vi "Compute Plot Legend Size.vi"(5 "# Plots":i32, 7 "Current Plot (Last)":i32=2147483647, 9 "Max Legend Size":i32) -> (6 "LegNumRows":u32, 8 "LegScrollVis":bool, 10 "LegScrollPos":u32)   [LabVIEW 2021, in "Graphs.lvlib"]
uses:
  Graphs.lvlib
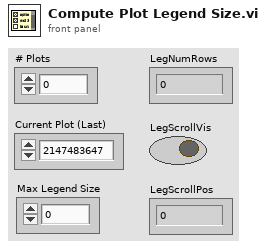
[diagram p1: front panel]
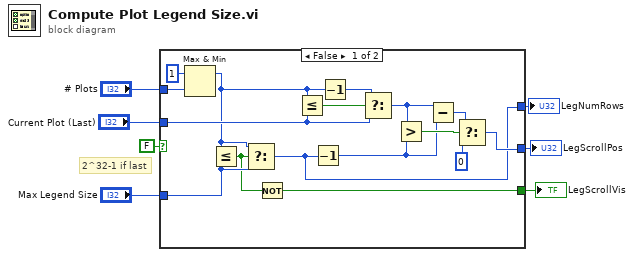
[diagram p0: block diagram]
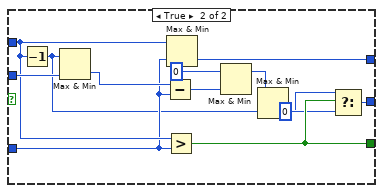
[diagram p2: hidden frame]
diagram:
  # "2^32-1 if last"
  n1 = case shown="False" FALSE {
    tunnel: [w8 w36] -> w7
    tunnel: [w9 w35] -> w6
    tunnel: [w12 w33] -> w5
    tunnel: "Current Plot (Last)" -> [w21 w32]
    tunnel: "# Plots" -> [w19 w31]
    tunnel: "Max Legend Size" -> [w16 w29]
    frame False {
      n2 = Max & Min(x=1, y=w19) -> (max(x,y)=w17:i32)  [unwired: 1 out]
      n3 = Less Or Equal?(x=w17, y=w16) -> (x <= y?=w10:bool)
      n4 = Select(t=w17, s=w10, f=w16) -> (s? t:f=w8:i32)
      n5 = Not(x=w10) -> (.not. x?=w9:bool)
      n6 = Less Or Equal?(x=w17, y=w21) -> (x <= y?=w23:bool)
      n7 = Decrement(x=w8) -> (x-1=w11:i32)
      n8 = Decrement(x=w17) -> (x-1=w22:i32)
      n9 = Select(t=w22, s=w23, f=w21) -> (s? t:f=w15:i32)
      n10 = Greater?(x=w15, y=w11) -> (0:w20:bool)
      n11 = Subtract(x=w15, y=w11) -> (x-y=w14:i32)
      n12 = Select(t=w14, s=w20, f=0) -> (s? t:f=w12:i32)
    }
    frame True {
      n13 = Decrement(x=w31) -> (x-1=w28:i32)
      n14 = Max & Min(x=w28, y=w32) -> (min(x,y)=w30:i32)  [unwired: 1 out]
      n15 = Subtract(x=w30, y=w29) -> (x-y=w24:i32)
      n16 = Greater?(x=w31, y=w29) -> (0:w35:bool)
      n17 = Max & Min(x=w31, y=w29) -> (min(x,y)=w36:i32)  [unwired: 1 out]
      n18 = Max & Min(x=0, y=w24) -> (max(x,y)=w25:i32)  [unwired: 1 out]
      n19 = Max & Min(x=w25, y=w28) -> (min(x,y)=w27:i32)  [unwired: 1 out]
      n20 = Select(t=w27, s=w35, f=u32 0) -> (s? t:f=w33:u32)
    }
  }
  "LegScrollPos" <- w5
  "LegScrollVis" <- w6
  "LegNumRows" <- w7
